vi "Control Globals RD v1.0.vi"() -> ()   [LabVIEW 2019]
panel:
  in  "Startup OK":bool
  in  "CT-EN0-1003":dbl=0.0023897901978790982
  in  "CT-EN0-1002":dbl=0.0030660219635462336
  in  "CT-EN0-1001":dbl=0.0015053297855240665
  in  "Shutdown?":bool
  out "3p PTO1 Time Stamp":timestamp=timestamp(3711389663.5462666 s since 1904-01-01)
  in  "PT-EN0-1003 (rms)":dbl=0.0030419968691409007
  in  "PT-EN0-1002 (rms)":dbl=0.0026653398841474953
  in  "PT-EN0-1001 (rms)":dbl=0.006708184020763715
  # "PTs"
  # "CTs"
  # "HMI User Input"
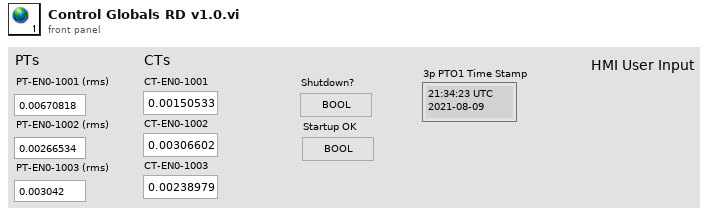
[diagram p1: front panel]
diagram:
